vi "ProjectRun.vi"(8 "error in (no error)":errorcluster, 11 "Project.lvclass In":refnum<class "Project.lvclass">) -> (0 "error out":errorcluster, 1 "VirtualDataArray":refnum<class "VirtualOrigin.lvclass">[](array[class]), 2 "StepDataArray":refnum<class "StepData.lvclass">[](array[class]), 3 "Project.lvclass Out":refnum<class "Project.lvclass">)   [LabVIEW 2014, in "Project.lvclass"]
uses:
  Project.lvclass
  StepData/StepData.lvclass
  Virtual/VirtualOrigin.lvclass
  Project.lvclass/Project.ctl
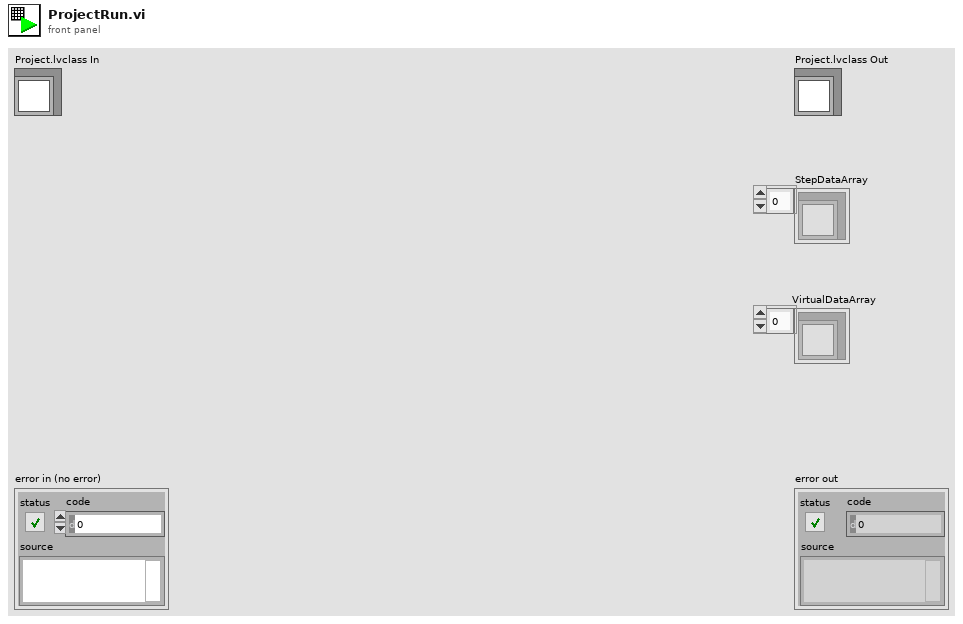
[diagram p1: front panel]
types:
  T1 = typedef "Project.lvclass/ProjectDataTableTypeDefine.ctl" = string[][]
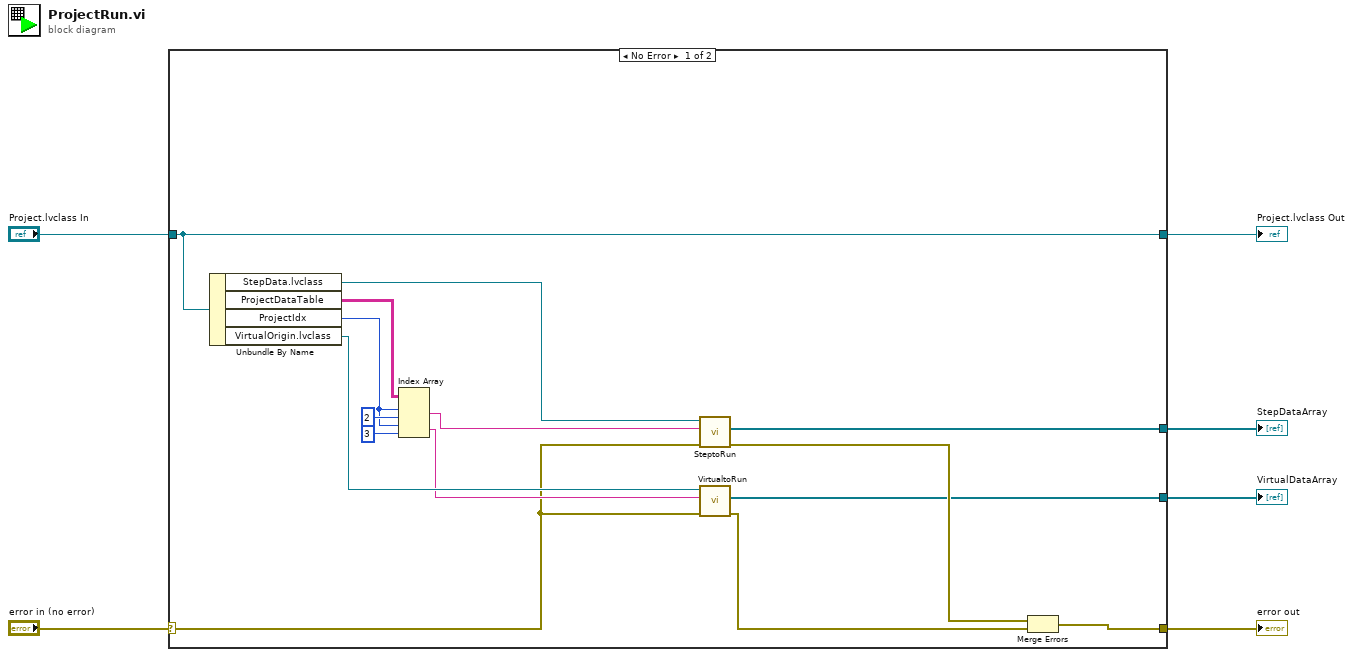
[diagram p0: block diagram]
diagram:
  n1 = case shown="No Error" "error in (no error)" {
    selector: "error in (no error)" -> [w9 w23]
    tunnel: [w19 w23] -> w5
    tunnel: "Project.lvclass In" -> [w18 w22]
    tunnel: [w18 w22] -> w3
    tunnel: [w15 _] -> w2
    tunnel: [w7 _] -> w1
    frame No Error {
      n2 = Unbundle By Name(w18) -> ("StepData.lvclass"=w17:refnum<class "StepData.lvclass">, "ProjectDataTable"=w21:T1, "ProjectIdx"=w11:i32, "VirtualOrigin.lvclass"=w13:refnum<class "VirtualOrigin.lvclass">)
      n3 = Index Array(array=w21, index (row) #1=w11, index (col) #1=2 ("disabled index (col)"), index (row) #2=w11, index (col) #2=3 ("index (col)")) -> (element #1=w16:string, element #2=w10:string)
      n4 = call "SteptoRun.vi"("error in (no error)"=w9, "StepSetup"=w16, "StepData.lvclass In"=w17) -> ("error out"=w14:errorcluster, "StepDataArray"=w15:refnum<class "StepData.lvclass">[])  [unwired: 7 in]
      n5 = call "VirtualtoRun.vi"("error in (no error)"=w9, "VirtualSetup"=w10, "VirtualOrigin.lvclass In"=w13) -> ("error out"=w8:errorcluster, "VirtualDataArray"=w7:refnum<class "VirtualOrigin.lvclass">[])  [unwired: 7 in]
      n6 = Merge Errors(w14, w8) -> (w19:errorcluster)
    }
    frame Error {
    }
  }
  "error out" <- w5
  "Project.lvclass Out" <- w3
  "StepDataArray" <- w2
  "VirtualDataArray" <- w1
